vi "Examples Images2.vi"() -> ()   [LabVIEW 2020, in "LcPictureBox.lvclass"]
uses:
  <userlib>/_LabVIEWCommon/LcPictureBox_class/LcPictureBox.lvclass
  <userlib>/_LabVIEWCommon/LcPictureBox_class/Pen.ctl
  <userlib>/_LabVIEWCommon/LcPictureBox_class/LcPictureBox.lvclass/LcPictureBox.ctl
  System.Windows.Forms
panel:
  in  "Rotation(0deg)":dbl=45.0 format="%#_13g"
  in  "ImageOffset":cluster{"x":sgl, "y":sgl}={"x"=-96.0, "y"=-333.0}
  out "Error Out":errorcluster
  in  "PictureBox":refnum<k24>(container)
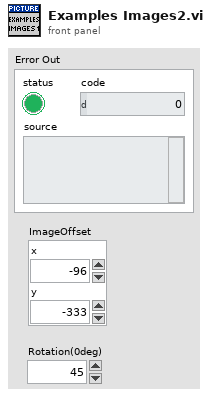
[diagram p1: front panel]
types:
  T1 = typedef "LcPictureBox.lvclass/Pen.ctl" = cluster{"Width":dbl, "Style":enum32{"Solid", "Dash", "Dot", "DashDot", "DashDotDot"}}
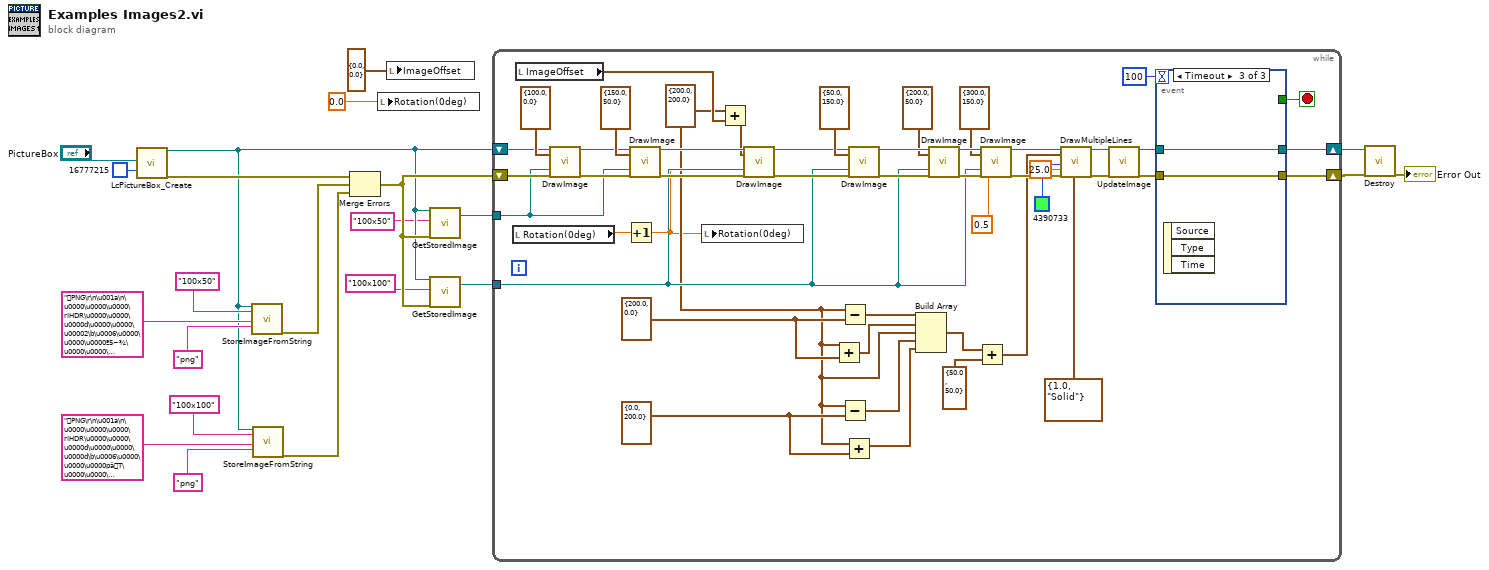
[diagram p0: block diagram]
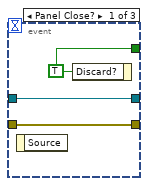
[diagram p2: hidden frame]
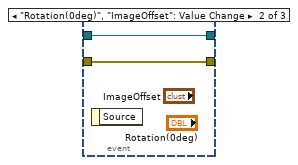
[diagram p3: hidden frame]
diagram:
  n1 = call <userlib>:"LcPictureBox_Create.vi"("PictureBox"="PictureBox", "BgColor(None)"=u32 16777215) -> ("reference out"=w7:refnum<class "LcPictureBox.lvclass">, "Error Out"=w17:errorcluster)  [unwired: 15 in, 1 out]
  n2 = call <userlib>:"StoreImageFromString.vi"("reference in"=w7, "ImageName"="100x50", "ImageFileContent"="PNG\r\n\u001a\n\u0000\u0000\u0000\rIHDR\u0000\u0000\u0000d\u0000\u0000\u00002\b\u0006\u0000\u0000\u0000ª5~¾\u0000\u0000\u0001iCCPICC profile\u0000\u0000(};HÃ@\u001cÆ¿¦\u000f*\nv\u0010QÈP,øB\u001c¥E°PÚ\n­:\\ú&\rI£àZpð±XupqÖÕÁU\u0010\u0004\u001f NN.RâÿB\u0018\u000fûñÝ}\u001fwß\u0001B­ÄT³m\u001cP5ËHD#b:³*v¼B@\u001fº0\tz,¹çøº¯waå}îÏÑ£dM\u0006øDâ9¦\u001b\u0016ñ\u0006ñÌ¦¥sÞ'\u000e²¤\u0010\u0013\u0019tAâG®Ë.¿qÎ;,ðÌ JÌ\u0013\u0007Å|\u000bË-Ì\nJ<M\u001cRTò´Ë\nç-Îj©Â\u001a÷ä/\fdµ$×i\u000e!%Ä\u0010\b\u0019\u0015\u0014Q0­\u001a)&\u0012´\u001fñð\u000f:þ8¹dr\u0015ÁÈ±2TH\u001fü\u000f~wkæ¦&Ý¤@\u0004h±í\u0011 c\u0017¨WmûûØ¶ë'ÿ\u0019¸Òþr\rý$½ÚÔBG@ï6pqÝÔä=àr\u0007\u0018xÒ%Cr$?M!\u0003ÞÏè2@ÿ-Ð½æöÖØÇé\u0003¢®oC`4OÙë\u001eïîlííß3þ~\u0000QrµKï\u0017d\u0000\u0000\u0000\u0006bKGD\u0000\u0000\u0000\u0000\u0000\u0000ùC»\u0000\u0000\u0000\tpHYs\u0000\u0000.#\u0000\u0000.#\u0001x¥?v\u0000\u0000\u0000\u0007tIME\u0007æ\u0002\u0010\t\u001f\u000bsIºY\u0000\u0000\u0000\u0019tEXtComment\u0000Created with GIMPW\u000e\u0017\u0000\u0000\u0003wIDATxÚí?Hrm\u0018Æ/¿h\u0012¡ÉI(\u001cB\u001c\u001a Z\u001a\"\u001aZF\u001b\"hijHj)rt$Z*§\u0004!\u001bª¡ì/EhsQ..." ("ImageFileFileExtention(png,jpg,...)"), "ImageFileFileExtention(png,jpg,...)"="png") -> ("error out"=w10:errorcluster)  [unwired: 14 in, 1 out]
  n3 = call <userlib>:"StoreImageFromString.vi"("reference in"=w7, "ImageName"="100x100", "ImageFileContent"="PNG\r\n\u001a\n\u0000\u0000\u0000\rIHDR\u0000\u0000\u0000d\u0000\u0000\u0000d\b\u0006\u0000\u0000\u0000pâT\u0000\u0000\u0001iCCPICC profile\u0000\u0000(ÏK(DQ\u001cÆîGDDÝ\u0005VW²Ô\u0010)Jc×Â½wÌPs¯éÞ¥²²ðØx-l¬ÙZØ*¥<JVVÄFºþçIrêt~}ç|_ç|\u0007´e{¥`;\u00197:\u0012Ñ§gfõòg4ê¨¤.ÃòÒãÃ1[JÔzÓ¡²øß¨/z\u0016èÂ\u0003VÚÍ\b/\b÷­eÒwÃÖ\u0011\u0017>\u0015nwåÂ÷J7sü¢8\u0019°¦2Ãn,:(\u001c\u0016Ö\u0005l\u0016°µäÚÂ½Â-qÛ|m:ÇqÅëíÔªõsOõÂêEgjRé2\u0018aq&Ð1Ye\u0014\u0019:duDñÊ~¤¿1ðOË\u0014×28XÁÆ\bü¨?øÝ­èéÎ%UG ìÉ÷ßZ¡|\u000b¾²¾ÿyèû_G\u0010z\u000b'ï_9þwÑ³y­e\u001fj7àì2¯Ûp¾\t\r\u000fiÃ5\u0002)$SK$àõD¾i\u0006ê¯¡j.×ÛÏ>Çw\u0010®Æ®`w\u000fÚ=_äÝ\u0015½ýy&èÈ7Qrµü\t=H\u0000\u0000\u0000\tpHYs\u0000\u0000\u000eÄ\u0000\u0000\u000eÄ\u0001+\u000e\u001b\u0000\u0000\u0000\u0006bKGD\u0000\u0000\u0000\u0000\u0000\u0000ùC»\u0000\u0000\u0000\u0007tIME\u0007æ\u0002\u0010\t\u001f9»ëÙ\u0000\u0000\u0000\u0019tEXtComment\u0000Created with GIMPW\u000e\u0017\u0000\u0000\u00077IDATx^íIh\u0014M\u0014Ç_Ü\u000f®|.\u0007sð³ \u0010ð&\b\"\"\"\"H\\¢¨ \u001eâv\u0013!\b\"^\\\u000e\"*\u00015n\u0018ô (\u0006\u0015\u0014½¸á\u0007=\u0005A..." ("ImageFileFileExtention(png,jpg,...)"), "ImageFileFileExtention(png,jpg,...)"="png") -> ("error out"=w9:errorcluster)  [unwired: 14 in, 1 out]
  n4 = Merge Errors(w17, w10, w9) -> (w8:errorcluster)
  n5 = local write "Rotation(0deg)"(0.0 ("Rotation(0deg)")) -> ()
  n6 = local write "ImageOffset"(cluster{"x":sgl, "y":sgl} {"x"=0.0, "y"=0.0} ("ImageOffset")) -> ()
  n7 = call-dynamic "GetStoredImage.vi"("reference in"=w7, "ImageName"="100x50", "error in (no error)"=w8) -> ("ImageOut"=w4:refnum<k24>)  [unwired: 13 in, 3 out]
  n8 = call-dynamic "GetStoredImage.vi"("reference in"=w7, "ImageName"="100x100", "error in (no error)"=w8) -> ("ImageOut"=w3:refnum<k24>)  [unwired: 13 in, 3 out]
  n9 = while {
    tunnel: w4 -> [w55]
    tunnel: w3 -> [w46]
    shift-right: [w64] -> w20
    shift-left: w8 -> [w57]
    shift-right: [w63] -> w19
    shift-left: w7 -> [w56]
    stop <- w30 stop-if-true
    w38 = cluster{"x":sgl, "y":sgl} {"x"=0.0, "y"=200.0} ("y")
    w43 = cluster{"x":sgl, "y":sgl} {"x"=200.0, "y"=0.0} ("y")
    w28 = cluster{"x":sgl, "y":sgl} {"x"=200.0, "y"=200.0} ("UpperLeftCorner")
    n10 = local read "Rotation(0deg)"() -> (w24:dbl)
    n11 = local read "ImageOffset"() -> (w29:cluster{"x":sgl, "y":sgl})
    n12 = call-dynamic "DrawImage.vi"("reference in"=w56, "UpperLeftCorner"=cluster{"x":sgl, "y":sgl} {"x"=100.0, "y"=0.0}, "Image"=w55, "Error In"=w57) -> ("reference out"=w59:refnum<class "LcPictureBox.lvclass">, "Error Out"=w58:errorcluster)  [unwired: 14 in]
    n13 = Increment(x=w24) -> (x+1=w23:dbl)
    n14 = call-dynamic "DrawImage.vi"("reference in"=w59, "UpperLeftCorner"=cluster{"x":sgl, "y":sgl} {"x"=150.0, "y"=50.0}, "Image"=w55, "Error In"=w58) -> ("reference out"=w50:refnum<class "LcPictureBox.lvclass">, "Error Out"=w49:errorcluster)  [unwired: 14 in]
    n15 = local write "Rotation(0deg)"(w23) -> ()
    n16 = Add(x=w28, y=w29) -> (x+y=w27:cluster{"x":sgl, "y":sgl})
    n17 = call-dynamic "DrawImage.vi"("reference in"=w50, "UpperLeftCorner"=w27, "Image"=w46, "Error In"=w49, "Rotation(0deg)"=w23) -> ("reference out"=w48:refnum<class "LcPictureBox.lvclass">, "Error Out"=w47:errorcluster)  [unwired: 13 in]
    n18 = Add(x=w28, y=w43) -> (x+y=w41:cluster{"x":sgl, "y":sgl})
    n19 = Subtract(x=w28, y=w43) -> (x-y=w42:cluster{"x":sgl, "y":sgl})
    n20 = Subtract(x=w28, y=w38) -> (x-y=w37:cluster{"x":sgl, "y":sgl})
    n21 = Add(x=w28, y=w38) -> (x+y=w36:cluster{"x":sgl, "y":sgl})
    n22 = call-dynamic "DrawImage.vi"("reference in"=w48, "UpperLeftCorner"=cluster{"x":sgl, "y":sgl} {"x"=50.0, "y"=150.0}, "Image"=w46, "Error In"=w47) -> ("reference out"=w67:refnum<class "LcPictureBox.lvclass">, "Error Out"=w66:errorcluster)  [unwired: 14 in]
    n23 = Build Array(w42, w41, w28, w37, w36) -> (w32:cluster{"x":sgl, "y":sgl}[])
    n24 = call-dynamic "DrawImage.vi"("reference in"=w67, "UpperLeftCorner"=cluster{"x":sgl, "y":sgl} {"x"=200.0, "y"=50.0}, "Image"=w46, "Error In"=w66) -> ("reference out"=w54:refnum<class "LcPictureBox.lvclass">, "Error Out"=w53:errorcluster)  [unwired: 14 in]
    n25 = Add(x=w32, y=cluster{"x":sgl, "y":sgl} {"x"=50.0, "y"=50.0}) -> (x+y=w31:cluster{"x":sgl, "y":sgl}[])
    n26 = call-dynamic "DrawImage.vi"("reference in"=w54, "UpperLeftCorner"=cluster{"x":sgl, "y":sgl} {"x"=300.0, "y"=150.0}, "Image"=w46, "Error In"=w53, "ScaleFactor(1)"=0.5) -> ("reference out"=w34:refnum<class "LcPictureBox.lvclass">, "Error Out"=w45:errorcluster)  [unwired: 13 in]
    n27 = call-dynamic "DrawMultipleLines.vi"("reference in"=w34, "LineEndPoints"=w31, "Color(Black)"=u32 4390733, "Alpha(100%)"=25.0, "Error In"=w45, "Pen(Width=1, Solid)"=T1 {"Width"=1.0, "Style"=enum."Solid"}) -> ("reference out"=w35:refnum<class "LcPictureBox.lvclass">, "Error Out"=w44:errorcluster)  [unwired: 12 in]
    n28 = call-dynamic "UpdateImage.vi"("reference in"=w35, "Error In"=w44) -> ("reference out"=w61:refnum<class "LcPictureBox.lvclass">, "Error Out"=w62:errorcluster)  [unwired: 14 in, 2 out]
    n29 = event shown="[2] Timeout" {
      selector: _ -> [_ _ _]
      dyn-events: _ -> [_ _ _]
      timeout: 100 -> [_ _ _]
      tunnel: w62 -> [w72 w73 w75]
      tunnel: [w72 w73 w75] -> w64
      tunnel: w61 -> [w71 w74 w76]
      tunnel: [w71 w74 w76] -> w63
      tunnel: [w70 _ _] -> w30
      event Panel Close? {
        w70 = TRUE ("Discard?")
        n30 = event-data() -> ()  [unwired: 1 in, 1 out]
        n31 = event-data("Discard?"=w70) -> ()  [unwired: 1 in, 1 out]
      }
      event "Rotation(0deg)", "ImageOffset": Value Change {
        n32 = event-data() -> ()  [unwired: 1 in, 1 out]
      }
      event Timeout {
        n33 = event-data() -> ()  [unwired: 1 in, 3 out]
      }
    }
  }
  n34 = call-dynamic "Destroy.vi"("reference in"=w19, "Error In"=w20) -> ("Error Out"=→"Error Out":errorcluster)  [unwired: 16 in, 1 out]
